vi "Laser Power Controller Control Panel (No Objects).vi"(8 "error in (no error)":errorcluster) -> (0 "error out":errorcluster)   [LabVIEW 2012]
doc: "(Dynamic) A user-level application that simulates the physical front panel of the Instrument. Provide the user with buttons to manually control features of the instrument, and provide indicators of its current state."
uses:
  <vilib>/Utility/error.llb/DialogType.ctl
  Power Meter/Newport 1830-C/Public/Filters.ctl
  BEOC LPC/BEOC LPC.lvlib
panel:
  in  "Power Meter\nVISA Resource Name":refnum<visa-resource-name>="GPIB0::4::INSTR"
  in  "Laser Power Controller\nVISA Resource Name":refnum<visa-resource-name>="GPIB0::3::INSTR"
  in  "Current Power\n(set by user)":dbl[unit]
  in  "Designate \nCurrent Power":bool
  in  "Filters":u16(ring)=3 items=["ND .1"=1, "ND .3"=3, "ND .5"=5, "ND 1"=10, "ND 2"=20, "ND 3"=30]
  in  "ND Filter?":bool
  out "Desired Power\nLoop Counter":i32
  in  "Timeout":i32=-1
  in  "Continuous Read":bool
  out "Transmission (%)":dbl format="%.2g"
  in  "transmission (%)":dbl=75.0 format="%.2g"
  in  "Set Transmission":bool
  in  "Set front-panel controls":bool
  in  "Set Control Mode":bool
  in  "Set Wavelength":bool
  in  "Set Power":bool
  out "Current Power\n(From Power Meter)":string caption="of Reflected Beam"
  in  "Read Power":bool
  in  "Go to Desired Power":bool
  in  "Desired Power":dbl[unit]
  in  "Configure Power Meter":bool
  in  "Read to Control":bool
  in  "Read":bool
  in  "Copy actual to set":bool
  in  "Populate fields with member data":bool
  out "Front-Panel Controls":enum16{"enabled", "disabled"}(ring)
  out "Control Mode":T1(ring)
  out "Wavelength":dbl[unit]
  out "Power":dbl[unit] format="%.2g"
  in  "front-panel controls":enum16{"enabled", "disabled"}(ring)
  in  "control mode":T1(ring)
  in  "wavelength":dbl[unit]=8.300000000000001e-07
  in  "power":dbl[unit]=0.005 format="%.2g"
  in  "stop":bool
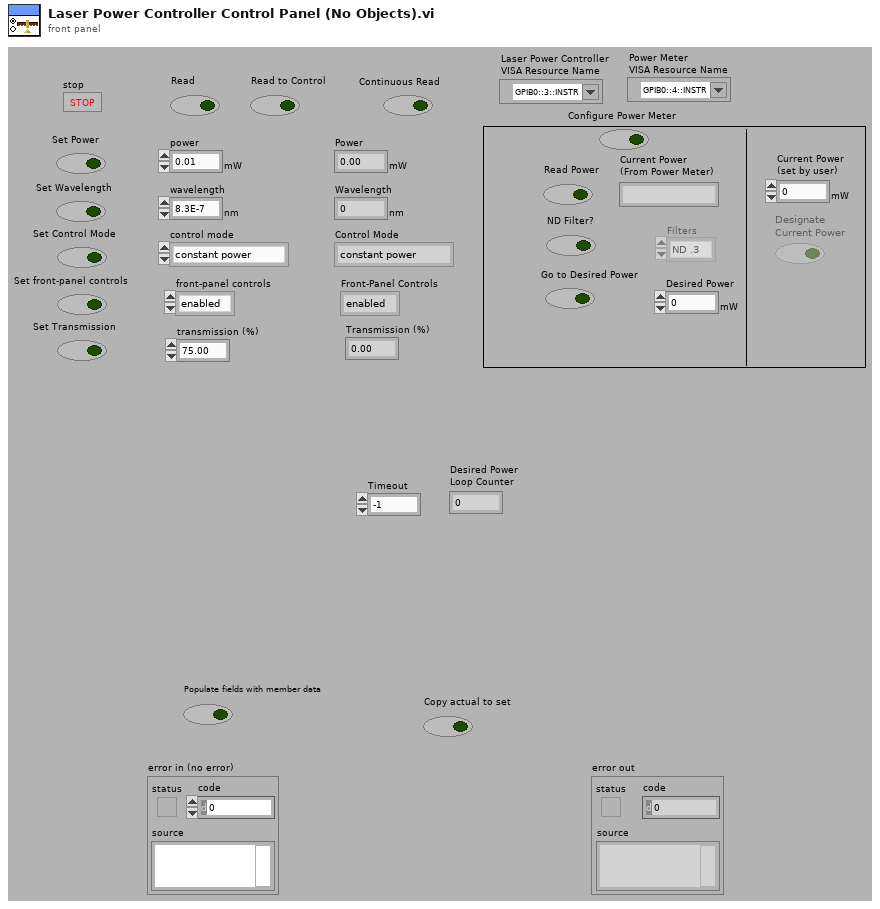
[diagram p1: front panel]
types:
  T1 = enum16{"constant power", "constant transmission"}
  T2 = cluster{"power":dbl[unit], "wavelength":dbl[unit], "control mode":enum16{"constant power", "constant transmission"}, "front-panel controls":enum16{"enabled", "disabled"}, "transmission (%)":dbl}
  T3 = typedef "Filters.ctl" = u16
  T4 = cluster{"Wavelength":dbl[unit], "AVG":u16, "Range":u16, "Backlight":u16, "Beeper":u16, "Zero":u16, "Local Lockout":u16, "ATTN":u16, "Run/Stop":u16, "Units":u16, "Averaging Time":dbl, "Averaging":bool, "Most Recent Power":dbl, "Filter":T3}
  T5 = enum8{"Enabled", "Disabled", "Disabled and Grayed Out"}
  T6 = typedef "DialogType.ctl" = u16
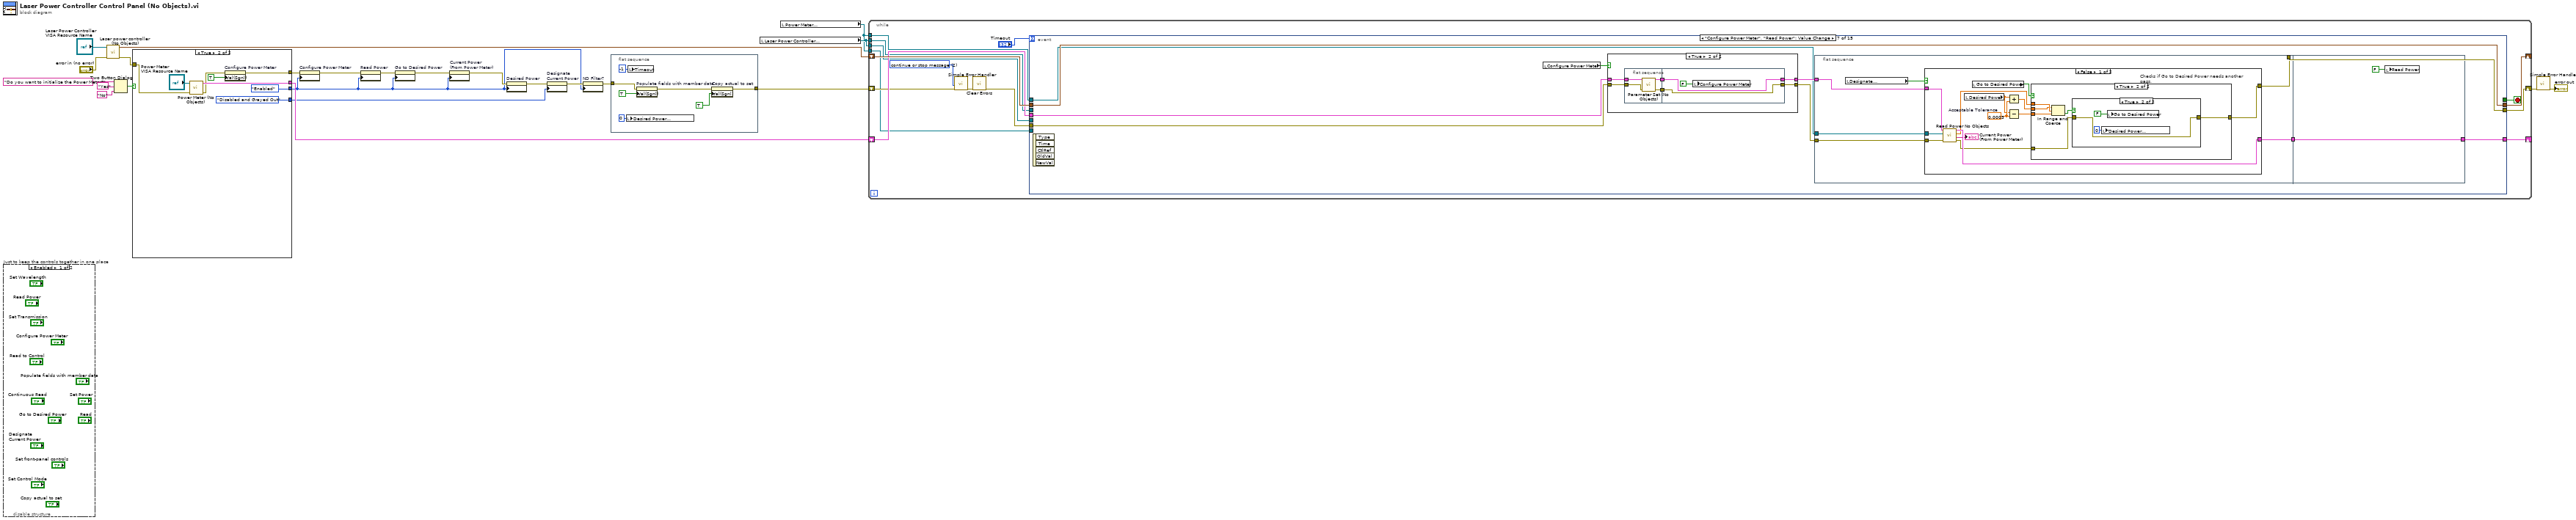
[diagram p0: block diagram]
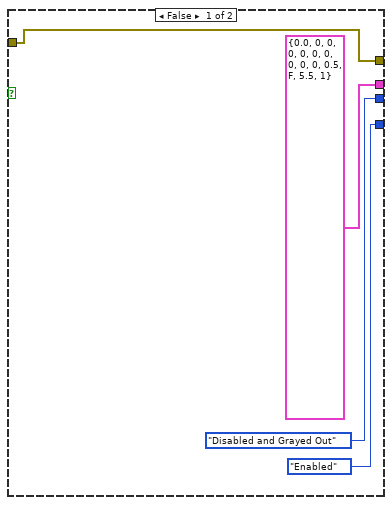
[diagram p2: hidden frame]
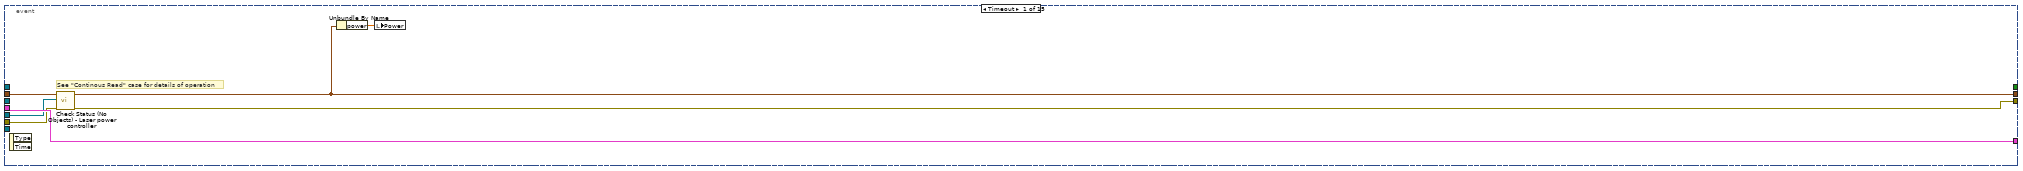
[diagram p4: hidden frame]
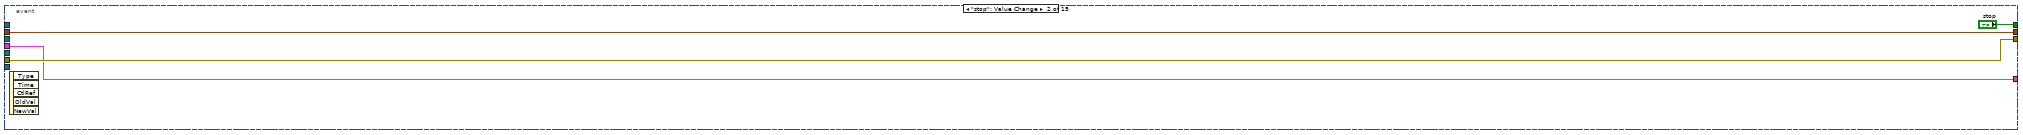
[diagram p5: hidden frame]
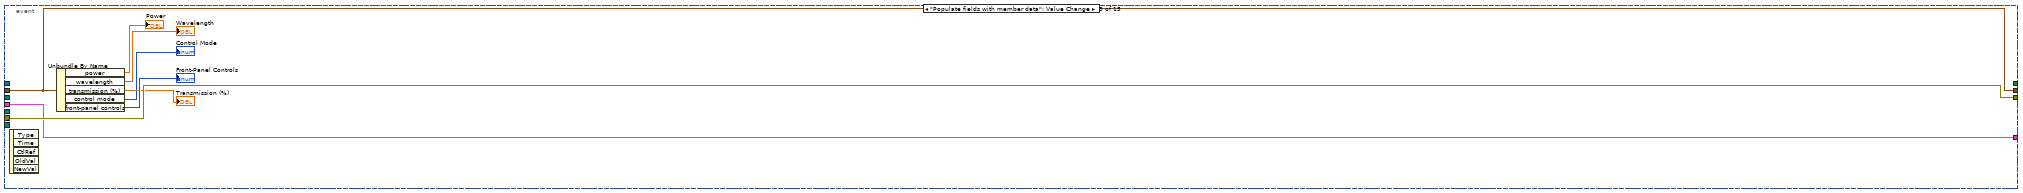
[diagram p6: hidden frame]
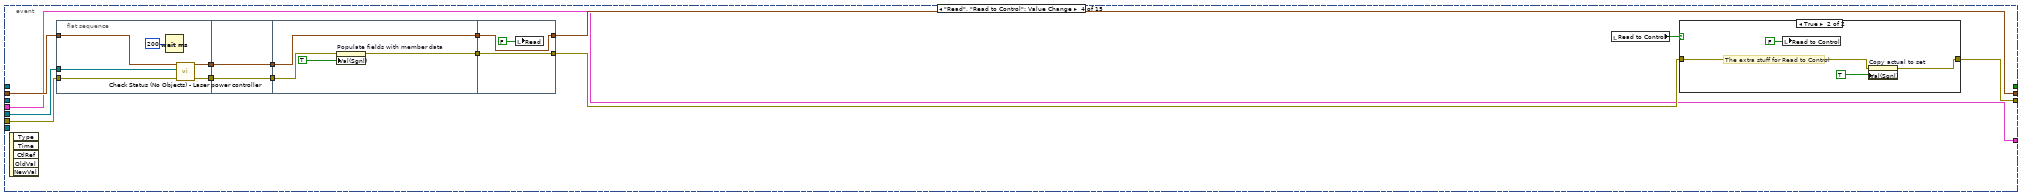
[diagram p7: hidden frame]
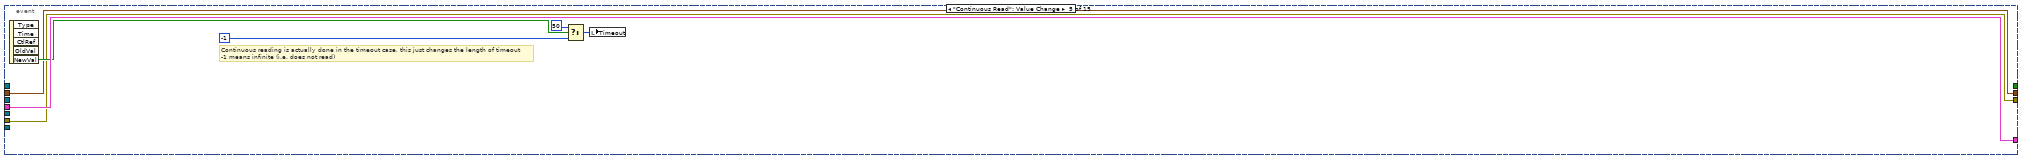
[diagram p9: hidden frame]
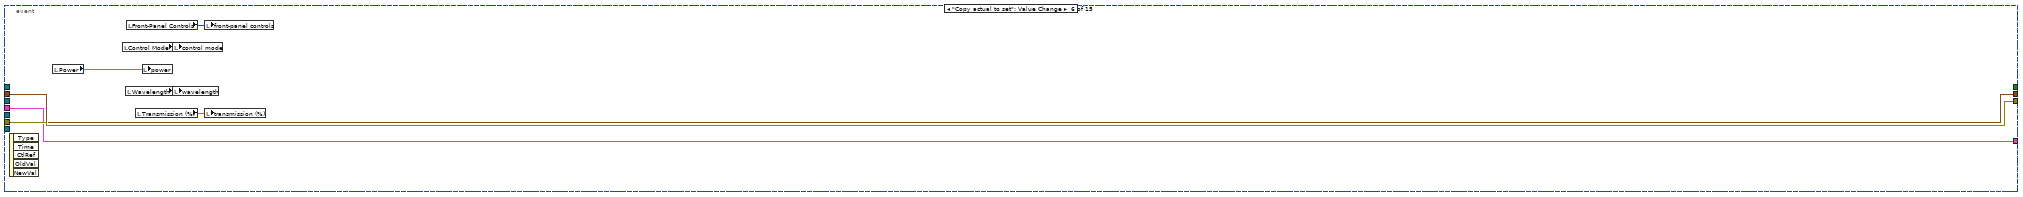
[diagram p10: hidden frame]
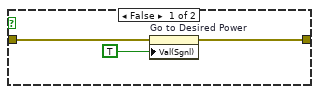
[diagram p12: hidden frame]
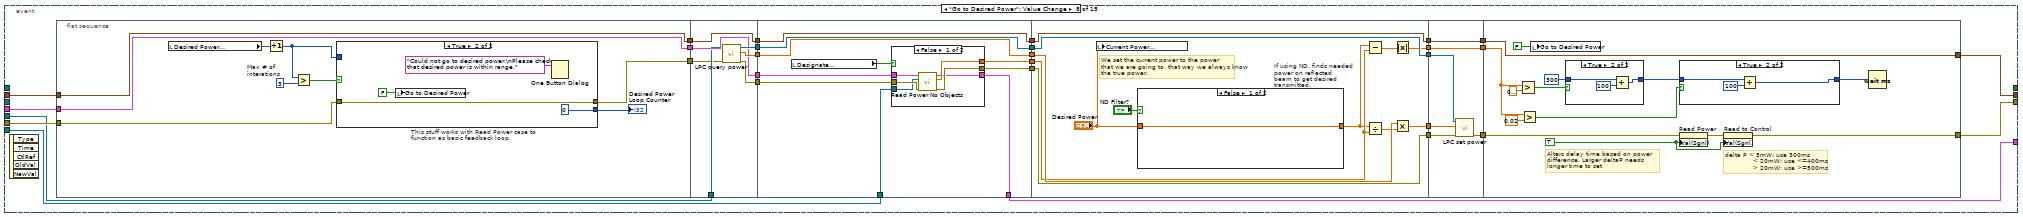
[diagram p15: hidden frame]
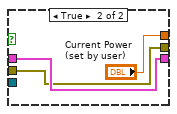
[diagram p17: hidden frame]
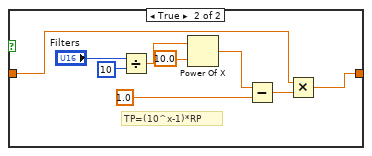
[diagram p18: hidden frame]
diagram:
  n1 = disable-structure "Just to keep the controls together in one place" shown="Enabled" {
    frame Enabled {
    }
    frame Disabled {
    }
  }
  n2 = call "Laser power controller (No Objects).vi"("error in (no error)"="error in (no error)", "VISA Resource Name"="Laser Power Controller\nVISA Resource Name") -> ("error out"=w5:errorcluster, "Cluster out"=w4:T2)  [unwired: 8 in]
  n3 = Two Button Dialog(message="Do you want to initialize the Power Meter?", 1:"No" ("F button name (\"Cancel\")"), 2:"Yes" ("T button name (\"OK\")")) -> (T button?=w9:bool)
  n4 = case shown="True" w9 {
    tunnel: w5 -> [w28 w31]
    tunnel: [T4 {"Wavelength"=0.0, "AVG"=0, "Range"=0, "Backlight"=0, "Beeper"=0, "Zero"=0, "Local Lockout"=0, "ATTN"=0, "Run/Stop"=0, "Units"=0, "Averaging Time"=0.5, "Averaging"=FALSE, "Most Recent Power"=5.5, "Filter"=1} ("Cluster of class private data") w32] -> w21
    tunnel: [w28 w35] -> w17
    tunnel: [T5."Disabled and Grayed Out" ("Disabled") T5."Enabled" ("Disabled")] -> w8
    tunnel: [T5."Enabled" ("Disabled") T5."Disabled and Grayed Out" ("Disabled")] -> w12
    frame False {
    }
    frame True {
      n5 = call "Power Meter (No Objects).vi"("error in (no error)"=w31, "VISA resource name"="Power Meter\nVISA Resource Name") -> ("error out"=w30:errorcluster, "Power Meter Out"=w32:T4)  [unwired: 8 in]
      n6 = property on="Configure Power Meter" class="Bool (strict)"(error in=w30, "Val(Sgnl)"=TRUE ("Value (Signaling)")) -> (error out=w35:errorcluster)  [unwired: 1 in, 1 out]
    }
  }
  n7 = property on="Configure Power Meter" class="Bool (strict)"(error in=w17, "DisabledEnum"=w8) -> (error out=w13:errorcluster)  [unwired: 1 in, 1 out]
  n8 = property on="Read Power" class="Bool (strict)"(error in=w13, "DisabledEnum"=w8) -> (error out=w16:errorcluster)  [unwired: 1 in, 1 out]
  n9 = property on="Go to Desired Power" class="Bool (strict)"(error in=w16, "DisabledEnum"=w8) -> (error out=w15:errorcluster)  [unwired: 1 in, 1 out]
  n10 = property on="Current Power\n(From Power Meter)" class="Str"(error in=w15, "DisabledEnum"=w8) -> (error out=w14:errorcluster)  [unwired: 1 in, 1 out]
  n11 = property on="Desired Power" class="DigNum (strict)"(error in=w14, "DisabledEnum"=w8) -> (error out=w10:errorcluster)  [unwired: 1 in, 1 out]
  n12 = property on="Designate \nCurrent Power" class="Bool (strict)"(error in=w10, "DisabledEnum"=w12) -> (error out=w11:errorcluster)  [unwired: 1 in, 1 out]
  n13 = property on="ND Filter?" class="Bool (strict)"(error in=w11, "DisabledEnum"=w8) -> (error out=w22:errorcluster)  [unwired: 1 in, 1 out]
  n14 = flat-sequence {
    tunnel: [w41] -> w24
    tunnel: w22 -> [w40]
    frame #0 {
      n15 = local write "Desired Power\nLoop Counter"(0 ("Desired Power\nLoop Counter")) -> ()
      n16 = local write "Timeout"(-1 ("Timeout")) -> ()
      n17 = property on="Populate fields with member data" class="Bool (strict)"(error in=w40, "Val(Sgnl)"=TRUE ("Value (Signaling)")) -> (error out=w43:errorcluster)  [unwired: 1 in, 1 out]
      n18 = property on="Copy actual to set" class="Bool (strict)"(error in=w43, "Val(Sgnl)"=TRUE ("Value (Signaling)")) -> (error out=w41:errorcluster)  [unwired: 1 in, 1 out]
    }
  }
  n19 = local read "Laser Power Controller\nVISA Resource Name"() -> (w2:refnum<visa-resource-name>)
  n20 = local read "Power Meter\nVISA Resource Name"() -> (w1:refnum<visa-resource-name>)
  n21 = while {
    shift-right: [w56] -> _
    shift-left: w4 -> [w57]
    shift-right: [w55] -> w23
    shift-left: w24 -> [w51]
    shift-right: [w53] -> _
    shift-left: w21 -> [w54]
    tunnel: w2 -> [w47]
    tunnel: w2 -> [w46]
    tunnel: w1 -> [w45]
    tunnel: w1 -> [w44]
    stop <- w58 stop-if-true
    w50 = T6 2 items=["no dialog", "OK message", "continue or stop message", "OK message + warnings", "continue/stop + warnings"] ("type of dialog (OK msg:1)")
    n22 = call <vilib>:"Simple Error Handler.vi"("type of dialog (OK msg:1)"=w50, "error in (no error)"=w51) -> ("error out"=w49:errorcluster)  [unwired: 3 in, 4 out]
    n23 = call <vilib>:"Clear Errors.vi"("error in (no error)"=w49) -> ("error out"=w48:errorcluster)  [unwired: 6 in]
    n24 = event shown="[6] \"Configure Power Meter\", \"Read Power\": Value Change" {
      selector: _ -> [_ _ _ _ _ _ _ _ _ _ _ _ _ _ _]
      dyn-events: _ -> [_ _ _ _ _ _ _ _ _ _ _ _ _ _ _]
      timeout: "Timeout" -> [_ _ _ _ _ _ _ _ _ _ _ _ _ _ _]
      tunnel: [_ "stop" _ _ _ _ _ _ _ _ _ _ _ _ _] -> w58
      tunnel: w57 -> [w61 w68 w76 w91 w112 w125 w136 w215 w315 w336 w354 w373 w391 w408 w417]
      tunnel: [w60 w68 w76 w90 w112 w125 w136 w209 w310 w331 w349 w369 w385 w408 w417] -> w56
      tunnel: w48 -> [w64 w67 w77 w87 w113 w126 w131 w214 w314 w335 w353 w372 w390 w405 w416]
      tunnel: [w62 w67 w77 w84 w113 w126 w128 w208 w309 w332 w351 w368 w387 w401 w409] -> w55
      tunnel: w54 -> [w65 w66 w73 w83 w118 w120 w130 w216 w313 w337 w355 w367 w389 _ _]
      tunnel: [w65 w66 w73 w83 w118 w120 w132 w191 w313 w337 w355 w367 w389 _ _] -> w53
      tunnel: w47 -> [w59 _ _ w78 _ _ _ w189 _ _ _ _ _ _ _]
      tunnel: w46 -> [_ _ _ _ _ _ _ _ w308 w330 w348 w366 w384 _ _]
      tunnel: w45 -> [_ _ _ _ _ _ w127 _ _ _ _ _ _ _ _]
      tunnel: w44 -> [_ _ _ _ _ _ _ w188 _ _ _ _ _ _ _]
      event Timeout {
        # "See \"Continous Read\" case for details of operation"
        n25 = event-data() -> ()  [unwired: 1 in, 2 out]
        n26 = call "Check Status (No Objects) - Laser power controller.vi"("error in (no error)"=w64, "VISA Resource Name"=w59, "Cluster In"=w61) -> ("error out"=w62:errorcluster, "Cluster Out"=w60:T2)  [unwired: 5 in, 2 out]
        n27 = Unbundle By Name(w60) -> ("power"=w63:dbl[unit])
        n28 = local write "Power"(w63) -> ()
      }
      event "stop": Value Change {
        n29 = event-data() -> ()  [unwired: 1 in, 5 out]
      }
      event "Populate fields with member data": Value Change {
        n30 = event-data() -> ()  [unwired: 1 in, 5 out]
        n31 = Unbundle By Name(w76) -> ("power"=→"Power":dbl[unit], "wavelength"=→"Wavelength":dbl[unit], "transmission (%)"=→"Transmission (%)":dbl, "control mode"=→"Control Mode":T1, "front-panel controls"=→"Front-Panel Controls":enum16{"enabled", "disabled"})
      }
      event "Read", "Read to Control": Value Change {
        n32 = event-data() -> ()  [unwired: 1 in, 5 out]
        n33 = flat-sequence {
          tunnel: w87 -> [w102]
          tunnel: w91 -> [w99]
          tunnel: [w98] -> w82
          tunnel: [w101] -> w80
          tunnel: w78 -> [w97]
          tunnel: w82 -> [w104]
          tunnel: [w104] -> w81
          tunnel: w80 -> [w103]
          tunnel: [w103] -> w79
          tunnel: [w106] -> w89
          tunnel: [w107] -> w85
          tunnel: w81 -> [w106]
          tunnel: w79 -> [w105]
          tunnel: [w111] -> w90
          tunnel: w89 -> [w111]
          tunnel: [w109] -> w86
          tunnel: w85 -> [w109]
          frame #0 {
            n34 = Wait (ms)(milliseconds to wait=u32 200) -> ()  [unwired: 1 out]
            n35 = call "Check Status (No Objects) - Laser power controller.vi"("error in (no error)"=w102, "VISA Resource Name"=w97, "Cluster In"=w99) -> ("error out"=w101:errorcluster, "Cluster Out"=w98:T2)  [unwired: 5 in, 2 out]
          }
          frame #1 {
          }
          frame #2 {
            n36 = property on="Populate fields with member data" class="Bool (strict)"(error in=w105, "Val(Sgnl)"=TRUE ("Value (Signaling)")) -> (error out=w107:errorcluster)  [unwired: 1 in, 1 out]
          }
          frame #3 {
            n37 = local write "Read"(FALSE ("Read")) -> ()
          }
        }
        n38 = local read "Read to Control"() -> (w88:bool)
        n39 = case shown="True" w88 {
          tunnel: w86 -> [w92 w94]
          tunnel: [w92 w93] -> w84
          frame False {
          }
          frame True {
            # "The extra stuff for Read to Control"
            n40 = local write "Read to Control"(FALSE ("Read to Control")) -> ()
            n41 = property on="Copy actual to set" class="Bool (strict)"(error in=w94, "Val(Sgnl)"=TRUE ("Value (Signaling)")) -> (error out=w93:errorcluster)  [unwired: 1 in, 1 out]
          }
        }
      }
      event "Continuous Read": Value Change {
        # "Continuous reading is actually done in the timeout case, this just changes the length of timeout\n-1 means infinite (i.e. does not read)"
        n42 = event-data() -> ("NewVal"=w115:bool)  [unwired: 1 in, 4 out]
        n43 = Select(t=50, s=w115, f=-1) -> (s? t:f=w116:i32)
        n44 = local write "Timeout"(w116) -> ()
      }
      event "Copy actual to set": Value Change {
        n45 = event-data() -> ()  [unwired: 1 in, 5 out]
        n46 = local read "Power"() -> (w124:dbl[unit])
        n47 = local read "Control Mode"() -> (w122:T1)
        n48 = local read "Wavelength"() -> (w123:dbl[unit])
        n49 = local read "Front-Panel Controls"() -> (w121:enum16{"enabled", "disabled"})
        n50 = local read "Transmission (%)"() -> (w119:dbl)
        n51 = local write "power"(w124) -> ()
        n52 = local write "control mode"(w122) -> ()
        n53 = local write "wavelength"(w123) -> ()
        n54 = local write "front-panel controls"(w121) -> ()
        n55 = local write "transmission (%)"(w119) -> ()
      }
      event "Configure Power Meter", "Read Power": Value Change {
        n56 = event-data() -> ()  [unwired: 1 in, 5 out]
        n57 = local read "Configure Power Meter"() -> (w135:bool)
        n58 = case shown="True" w135 {
          tunnel: w131 -> [w173 w180]
          tunnel: w130 -> [w174 w179]
          tunnel: [w174 w177] -> w133
          tunnel: [w173 w175] -> w134
          frame False {
          }
          frame True {
            n59 = flat-sequence {
              tunnel: w180 -> [w184]
              tunnel: w179 -> [w181]
              tunnel: [w183] -> w178
              tunnel: [w182] -> w176
              tunnel: w178 -> [w186]
              tunnel: [w186] -> w177
              tunnel: w176 -> [w185]
              tunnel: [w185] -> w175
              frame #0 {
                n60 = call "Parameter Set (No Objects).vi"("error in (no error)"=w184, "Cluster In"=w181) -> ("error out"=w182:errorcluster, "Cluster Out"=w183:T4)  [unwired: 8 in]
              }
              frame #1 {
                n61 = local write "Configure Power Meter"(FALSE ("Value (Signaling)")) -> ()
              }
            }
          }
        }
        n62 = flat-sequence {
          tunnel: [w142] -> w129
          tunnel: w134 -> [w140]
          tunnel: w133 -> [w141]
          tunnel: [w138] -> w128
          tunnel: w127 -> [w137]
          tunnel: [w172] -> w132
          tunnel: w129 -> [w172]
          frame #0 {
            n63 = local read "Designate \nCurrent Power"() -> (w139:bool)
            n64 = case shown="False" w139 {
              tunnel: w141 -> [w144 w170]
              tunnel: [w154 w170] -> w142
              tunnel: w140 -> [w155 w169]
              tunnel: [w145 w169] -> w138
              tunnel: w137 -> [w143 _]
              frame False {
                w151 = dbl[unit] 0.0003  # Acceptable Tolerance
                n65 = call "Read Power No Objects.vi"("error in (no error)"=w155, "VISA Resource Name"=w143, "Cluster In"=w144) -> ("error out"=w152:errorcluster, "Current Power w/ Units"=→"Current Power\n(From Power Meter)":string, "Current Power"=w148:dbl[unit], "Cluster Out"=w154:T4)  [unwired: 5 in]
                n66 = local read "Desired Power"() -> (w150:dbl[unit])
                n67 = local read "Go to Desired Power"() -> (w149:bool)
                n68 = Add(x=w150, y=w151) -> (x+y=w147:dbl[unit])
                n69 = Subtract(x=w150, y=w151) -> (x-y=w146:dbl[unit])
                n70 = case "Checks if Go to Desired Power needs another pass." shown="True" w149 {
                  tunnel: [w156 w161] -> w145
                  tunnel: w152 -> [w156 w160]
                  tunnel: w148 -> [_ w159]
                  tunnel: w147 -> [_ w158]
                  tunnel: w146 -> [_ w157]
                  frame False {
                  }
                  frame True {
                    n71 = In Range and Coerce(upper limit=w158, x=w159, lower limit=w157) -> (In Range?=w162:bool)  [unwired: 1 out]
                    n72 = case shown="True" w162 {
                      tunnel: [w165 w166] -> w161
                      tunnel: w160 -> [w163 w166]
                      frame False {
                        n73 = property on="Go to Desired Power" class="Bool (strict)"(error in=w163, "Val(Sgnl)"=TRUE) -> (error out=w165:errorcluster)  [unwired: 1 in, 1 out]
                      }
                      frame True {
                        n74 = local write "Desired Power\nLoop Counter"(0 ("Desired Power\nLoop Counter")) -> ()
                        n75 = local write "Go to Desired Power"(FALSE ("Go to Desired Power")) -> ()
                      }
                    }
                  }
                }
              }
              frame True {
                # "Forces a single pass if user designated the power"
              }
            }
          }
          frame #1 {
            n76 = local write "Read Power"(FALSE ("Value (Signaling)")) -> ()
          }
        }
      }
      event "Go to Desired Power": Value Change {
        n77 = event-data() -> ()  [unwired: 1 in, 5 out]
        n78 = flat-sequence {
          tunnel: w214 -> [w219]
          tunnel: w215 -> [w224]
          tunnel: w216 -> [w225]
          tunnel: [w225] -> w205
          tunnel: [w224] -> w204
          tunnel: [w218] -> w203
          tunnel: [w238] -> w200
          tunnel: [w237] -> w198
          tunnel: [w233] -> w195
          tunnel: w205 -> [w236]
          tunnel: w204 -> [w233]
          tunnel: w203 -> [w232]
          tunnel: [w236] -> w192
          tunnel: [w235] -> w190
          tunnel: w189 -> [w234]
          tunnel: w200 -> [w248]
          tunnel: [w248] -> w199
          tunnel: w198 -> [w247]
          tunnel: [w247] -> w197
          tunnel: [w245] -> w196
          tunnel: w195 -> [w246]
          tunnel: [w246] -> w194
          tunnel: [w241] -> w193
          tunnel: w192 -> [w244]
          tunnel: [w243] -> w191
          tunnel: w190 -> [w242]
          tunnel: w188 -> [w239]
          tunnel: [w269] -> w213
          tunnel: w199 -> [w269]
          tunnel: w197 -> [w266]
          tunnel: w196 -> [w263]
          tunnel: [w264] -> w212
          tunnel: [w268] -> w211
          tunnel: w194 -> [w268]
          tunnel: [w267] -> w210
          tunnel: w193 -> [w267]
          tunnel: [w261] -> w202
          tunnel: w213 -> [w285]
          tunnel: w212 -> [w283]
          tunnel: w211 -> [w280]
          tunnel: w210 -> [w284]
          tunnel: [w280] -> w207
          tunnel: [w281] -> w206
          tunnel: w202 -> [w282]
          tunnel: [w282] -> w201
          tunnel: [w298] -> w208
          tunnel: [w299] -> w209
          tunnel: w207 -> [w299]
          tunnel: w206 -> [w295]
          tunnel: w201 -> [w287]
          frame #0 {
            w222 = 3  # Max # of interations
            n79 = local read "Desired Power\nLoop Counter"() -> (w223:i32)
            n80 = Increment(x=w223) -> (x+1=w220:i32)
            n81 = Greater?(x=w220, y=w222) -> (0:w221:bool)
            n82 = case "This stuff works with Read Power case to function as basic feedback loop." shown="True" w221 {
              tunnel: w220 -> [w226 _]
              tunnel: w219 -> [w227 w228]
              tunnel: [w227 w228] -> w218
              tunnel: [w226 0] -> w217
              frame False {
              }
              frame True {
                n83 = local write "Go to Desired Power"(FALSE ("Go to Desired Power")) -> ()
                n84 = One Button Dialog(message="Could not go to desired power.\nPlease check that desired power is within range." ("error source (\" \")")) -> ()  [unwired: 1 in, 1 out]
              }
            }
            "Desired Power\nLoop Counter" <- w217
          }
          frame #1 {
            n85 = call "LPC query power.vi"("error in (no error)"=w232, "VISA resource name"=w234) -> ("error out"=w235:errorcluster, "power"=w237:dbl[unit], "VISA resource name out"=w238:refnum<visa-resource-name>)  [unwired: 7 in]
          }
          frame #2 {
            n86 = local read "Designate \nCurrent Power"() -> (w240:bool)
            n87 = case shown="False" w240 {
              tunnel: [w254 "Current Power\n(set by user)"] -> w245
              tunnel: w244 -> [w250 w257]
              tunnel: [w251 w257] -> w243
              tunnel: w242 -> [w252 w256]
              tunnel: [w253 w256] -> w241
              tunnel: w239 -> [w249 _]
              frame False {
                n88 = call "Read Power No Objects.vi"("error in (no error)"=w252, "VISA Resource Name"=w249, "Cluster In"=w250) -> ("error out"=w253:errorcluster, "Current Power"=w254:dbl[unit], "Cluster Out"=w251:T4)  [unwired: 5 in, 1 out]
              }
              frame True {
              }
            }
          }
          frame #3 {
            # "We set the current power to the power\nthat we are going to, that way we always know\nthe true power."
            n89 = local write "Current Power\n(set by user)"("Desired Power") -> ()
            n90 = case "If using ND, finds needed power on reflected\nbeam to get desired transmitted." shown="False" "ND Filter?" {
              tunnel: [w270 w271] -> w260
              tunnel: "Desired Power" -> [w270 w272]
              frame False {
              }
              frame True {
                # "TP=(10^x-1)*RP"
                n91 = Divide(x="Filters", y=u16 10) -> (x/y=w273:dbl)
                n92 = Power Of X(1:10.0 ("x"), 2:w273) -> (0:w276:dbl)
                n93 = Subtract(x=w276, y=1.0) -> (x-y=w277:dbl)
                n94 = Multiply(x=w272, y=w277) -> (x*y=w271:dbl[unit])
              }
            }
            n95 = Subtract(x=w260, y=w263) -> (x-y=w262:dbl[unit])
            n96 = Divide(x=w260, y=w263) -> (x/y=w265:dbl)
            n97 = Absolute Value(x=w262) -> (abs(x)=w261:dbl[unit])
            n98 = Multiply(x=w266, y=w265) -> (x*y=w264:dbl[unit])
          }
          frame #4 {
            n99 = call "LPC set power.vi"("error in (no error)"=w284, "power"=w283, "VISA resource name"=w285) -> ("error out"=w281:errorcluster)  [unwired: 7 in, 1 out]
          }
          frame #5 {
            w296 = TRUE ("Value (Signaling)")
            # "Alters delay time based on power \ndifference. Larger deltaP needs\nlonger time to set"
            # "delta P < 5mW: use 300ms\n              < 20mW: use <=400ms\n              > 20mW: use >=500ms"
            n100 = Greater?(x=w287, y=dbl[unit] 0.005) -> (0:w292:bool)
            n101 = Greater?(x=w287, y=dbl[unit] 0.02) -> (0:w290:bool)
            n102 = local write "Go to Desired Power"(FALSE ("Go to Desired Power")) -> ()
            n103 = case shown="True" w292 {
              tunnel: u32 300 ("Desired Power Delay") -> [w304 w307]
              tunnel: [w304 w305] -> w289
              frame False {
              }
              frame True {
                n104 = Add(x=w307, y=u32 100) -> (x+y=w305:u32)
              }
            }
            n105 = case shown="True" w290 {
              tunnel: w289 -> [w300 w302]
              tunnel: [w300 w301] -> w288
              frame False {
              }
              frame True {
                n106 = Add(x=w302, y=u32 100) -> (x+y=w301:u32)
              }
            }
            n107 = property on="Read Power" class="Bool (strict)"(error in=w295, "Val(Sgnl)"=w296) -> (error out=w297:errorcluster)  [unwired: 1 in, 1 out]
            n108 = property on="Read to Control" class="Bool (strict)"(error in=w297, "Val(Sgnl)"=w296) -> (error out=w298:errorcluster)  [unwired: 1 in, 1 out]
            n109 = Wait (ms)(milliseconds to wait=w288) -> ()  [unwired: 1 out]
          }
        }
      }
      event "Set Power": Value Change {
        n110 = event-data() -> ()  [unwired: 1 in, 5 out]
        n111 = flat-sequence {
          tunnel: w315 -> [w316]
          tunnel: w314 -> [w319]
          tunnel: [w317] -> w312
          tunnel: [w316] -> w311
          tunnel: w308 -> [w318]
          tunnel: w312 -> [w328]
          tunnel: w311 -> [w329]
          tunnel: [w329] -> w310
          tunnel: [w328] -> w309
          frame #0 {
            n112 = Add(x="power", y=dbl[unit] 0.00011899999999999999) -> (x+y=w323:dbl[unit])
            n113 = Divide(x=w323, y=1.0044) -> (x/y=w320:dbl[unit])
            n114 = call "LPC set power.vi"("error in (no error)"=w319, "power"=w320, "VISA resource name"=w318) -> ("error out"=w317:errorcluster)  [unwired: 7 in, 1 out]
          }
          frame #1 {
            n115 = local write "Set Power"(FALSE) -> ()
            n116 = Wait (ms)(milliseconds to wait=u32 500) -> ()  [unwired: 1 out]
            n117 = property on="Read" class="Bool (strict)"("Val(Sgnl)"=TRUE) -> ()  [unwired: 2 in, 2 out]
          }
        }
      }
      event "Set Wavelength": Value Change {
        n118 = event-data() -> ()  [unwired: 1 in, 5 out]
        n119 = flat-sequence {
          tunnel: w336 -> [w340]
          tunnel: w335 -> [w339]
          tunnel: [w341] -> w334
          tunnel: [w340] -> w333
          tunnel: w330 -> [w338]
          tunnel: w334 -> [w346]
          tunnel: w333 -> [w347]
          tunnel: [w347] -> w331
          tunnel: [w346] -> w332
          frame #0 {
            n120 = call "LPC set wavelength.vi"("error in (no error)"=w339, "wavelength"="wavelength", "VISA resource name"=w338) -> ("error out"=w341:errorcluster)  [unwired: 7 in, 1 out]
          }
          frame #1 {
            n121 = local write "Set Wavelength"(FALSE) -> ()
            n122 = Wait (ms)(milliseconds to wait=u32 100) -> ()  [unwired: 1 out]
            n123 = property on="Read" class="Bool (strict)"("Val(Sgnl)"=TRUE) -> ()  [unwired: 2 in, 2 out]
          }
        }
      }
      event "Set Transmission": Value Change {
        n124 = event-data() -> ()  [unwired: 1 in, 5 out]
        n125 = flat-sequence {
          tunnel: w354 -> [w357]
          tunnel: w353 -> [w359]
          tunnel: [w358] -> w352
          tunnel: [w357] -> w350
          tunnel: w348 -> [w356]
          tunnel: w352 -> [w365]
          tunnel: [w365] -> w351
          tunnel: w350 -> [w364]
          tunnel: [w364] -> w349
          frame #0 {
            n126 = call "LPC set transmission.vi"("error in (no error)"=w359, "transmission (%)"="transmission (%)", "VISA resource name"=w356) -> ("error out"=w358:errorcluster)  [unwired: 7 in, 1 out]
          }
          frame #1 {
            n127 = local write "Set Transmission"(FALSE) -> ()
            n128 = Wait (ms)(milliseconds to wait=u32 500) -> ()  [unwired: 1 out]
            n129 = property on="Read" class="Bool (strict)"("Val(Sgnl)"=TRUE) -> ()  [unwired: 2 in, 2 out]
          }
        }
      }
      event "Set Control Mode": Value Change {
        n130 = event-data() -> ()  [unwired: 1 in, 5 out]
        n131 = flat-sequence {
          tunnel: w373 -> [w375]
          tunnel: w372 -> [w374]
          tunnel: [w375] -> w371
          tunnel: [w376] -> w370
          tunnel: w366 -> [w377]
          tunnel: w371 -> [w382]
          tunnel: w370 -> [w383]
          tunnel: [w383] -> w368
          tunnel: [w382] -> w369
          frame #0 {
            n132 = call "LPC set control mode.vi"("error in (no error)"=w374, "control mode"="control mode", "VISA resource name"=w377) -> ("error out"=w376:errorcluster)  [unwired: 7 in, 1 out]
          }
          frame #1 {
            n133 = local write "Set Control Mode"(FALSE) -> ()
            n134 = Wait (ms)(milliseconds to wait=u32 100) -> ()  [unwired: 1 out]
            n135 = property on="Read" class="Bool (strict)"("Val(Sgnl)"=TRUE) -> ()  [unwired: 2 in, 2 out]
          }
        }
      }
      event "Set front-panel controls": Value Change {
        n136 = event-data() -> ()  [unwired: 1 in, 5 out]
        n137 = flat-sequence {
          tunnel: w391 -> [w394]
          tunnel: w390 -> [w392]
          tunnel: [w393] -> w388
          tunnel: [w394] -> w386
          tunnel: w384 -> [w395]
          tunnel: w388 -> [w400]
          tunnel: [w400] -> w387
          tunnel: w386 -> [w399]
          tunnel: [w399] -> w385
          frame #0 {
            n138 = call "LPC set remote.vi"("error in (no error)"=w392, "front-panel controls"="front-panel controls", "VISA resource name"=w395) -> ("error out"=w393:errorcluster)  [unwired: 7 in, 1 out]
          }
          frame #1 {
            n139 = local write "Set front-panel controls"(FALSE) -> ()
            n140 = property on="Read" class="Bool (strict)"("Val(Sgnl)"=TRUE) -> ()  [unwired: 2 in, 2 out]
          }
        }
      }
      event "ND Filter?": Value Change {
        n141 = event-data() -> ("NewVal"=w403:bool)  [unwired: 1 in, 4 out]
        n142 = Select(t=T5."Enabled" ("Disabled"), s=w403, f=T5."Disabled and Grayed Out" ("Disabled")) -> (s? t:f=w404:T5)
        n143 = property on="Filters" class="Ring (strict)"(error in=w405, "DisabledEnum"=w404) -> (error out=w402:errorcluster)  [unwired: 1 in, 1 out]
        n144 = property on="Current Power\n(From Power Meter)" class="Str"(error in=w402, "Caption.Visible"=w403) -> (error out=w401:errorcluster)  [unwired: 1 in, 1 out]
      }
      event "Designate \nCurrent Power": Value Change {
        n145 = event-data() -> ("NewVal"=w415:bool)  [unwired: 1 in, 4 out]
        n146 = Select(t=T5."Enabled" ("Disabled"), s=w415, f=T5."Disabled and Grayed Out" ("Disabled")) -> (s? t:f=w411:T5)
        n147 = property on="Current Power\n(set by user)" class="DigNum (strict)"(error in=w416, "DisabledEnum"=w411) -> (error out=w412:errorcluster)  [unwired: 1 in, 1 out]
        n148 = property on="Go to Desired Power" class="Bool (strict)"(error in=w412, "DisabledEnum"=w411) -> (error out=w410:errorcluster)  [unwired: 1 in, 1 out]
        n149 = property on="Desired Power" class="DigNum (strict)"(error in=w410, "DisabledEnum"=w411) -> (error out=w409:errorcluster)  [unwired: 1 in, 1 out]
      }
    }
  }
  n150 = call <vilib>:"Simple Error Handler.vi"("error in (no error)"=w23) -> ("error out"=→"error out":errorcluster)  [unwired: 1 in, 7 out]
